vi "Get remaining time.vi"(10 "Stop time":timestamp, 11 "Curent time":timestamp) -> (3 "Remaining time":string)   [LabVIEW 2020, in "UI.lvlib"]
uses:
  UI.lvlib
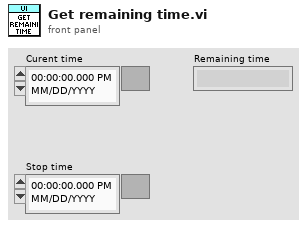
[diagram p1: front panel]
types:
  T1 = typedef "LVDateTimeRec.ctl" = cluster{"fractional second":dbl, "second":i32, "minute":i32, "hour":i32, "day of month":i32, "month":i32, "year":i32, "day of week":i32, "day of year":i32, "DST":i32}
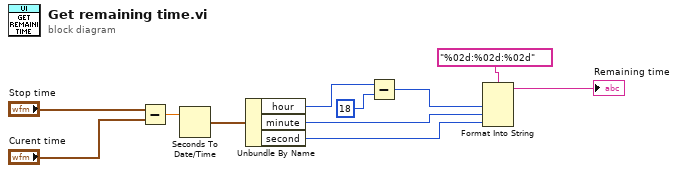
[diagram p0: block diagram]
diagram:
  n1 = Subtract(x="Stop time", y="Curent time") -> (x-y=w11:dbl)
  n2 = Seconds To Date/Time(time stamp (now)=w11) -> (date time rec=w8:T1)  [unwired: 1 in]
  n3 = Unbundle By Name(w8) -> ("hour"=w3:i32, "minute"=w6:i32, "second"=w5:i32)
  n4 = Subtract(x=w3, y=18) -> (x-y=w1:i32)
  n5 = Format Into String(format string="%02d:%02d:%02d" ("initial string"), w1, w6, w5) -> (resulting string=→"Remaining time":string)  [unwired: 2 in, 1 out]
